vi "CreateSetModeSoftAp Test.vi"() -> ()   [LabVIEW 2014, in "ESP8266 WiFi Wrapper.lvlib"]
uses:
  <vilib>/Aledyne-TSXperts/Arduino Compatible Compiler for LabVIEW/addons/ESP8266 WiFi Wrapper/ESP8266 WiFi Wrapper.lvlib
panel:
  in  "Listen Port":u8=80
  in  "WiFi Server Mode":T1(ring)=enum."WIFI_AP"
  in  "Password":string="at least 8 chars"
  in  "SSID":string="Library example name"
  out "Error Out":errorcluster
  in  "Error In":errorcluster
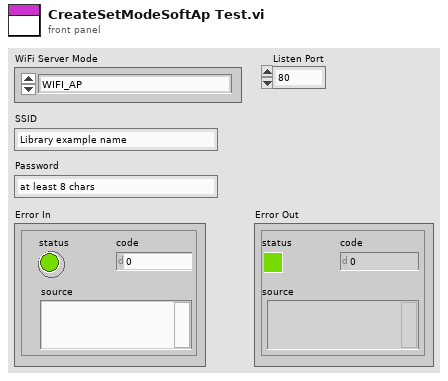
[diagram p1: front panel]
types:
  T1 = enum16{"WIFI_OFF", "WIFI_STA", "WIFI_AP", "WIFI_AP_STA"}
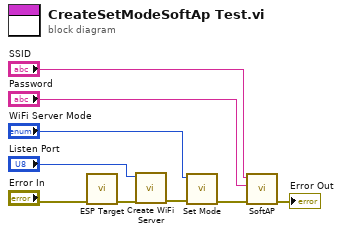
[diagram p0: block diagram]
diagram:
  n1 = call <vilib>:"ESP Target.vi"("Error In"="Error In") -> ("Error Out"=w2:errorcluster)  [unwired: 10 in]
  n2 = call <vilib>:"Create WiFi Server.vi"("Error In"=w2, "Listen Port"="Listen Port") -> ("Error Out"=w9:errorcluster)  [unwired: 9 in]
  n3 = call <vilib>:"Set Mode.vi"("Error In"=w9, "WiFi Server Mode"="WiFi Server Mode") -> ("Error Out"=w8:errorcluster)  [unwired: 9 in]
  n4 = call <vilib>:"SoftAP.vi"("Error In"=w8, "Password"="Password", "SSID"="SSID") -> ("Error Out"=→"Error Out":errorcluster)  [unwired: 8 in]
